vi "GUI_001.vi"(2 "Input":dbl) -> (0 "Slide":dbl(slide) scale=0.0..100.0)   [LabVIEW 2019]
doc: "This VI adds noise to user defined data"
uses:
  <vilib>/Analysis/baseanly.llb/Mean (DBL).vi
  <vilib>/Analysis/NI_AALBase.lvlib
panel:
  out "Histogram Graph":T1(graph)
  out "output data mean":dbl format="%0.2f"
  out "Output data":dbl[](array[numeric])
  in  "noise offset":dbl
  in  "noise gain":dbl
  in  "Operation Menu":T2(ring)
  out "Indicator":string
  in  "Control":string
  in  "stop":bool
  out "Waveform Chart":dbl(graph)
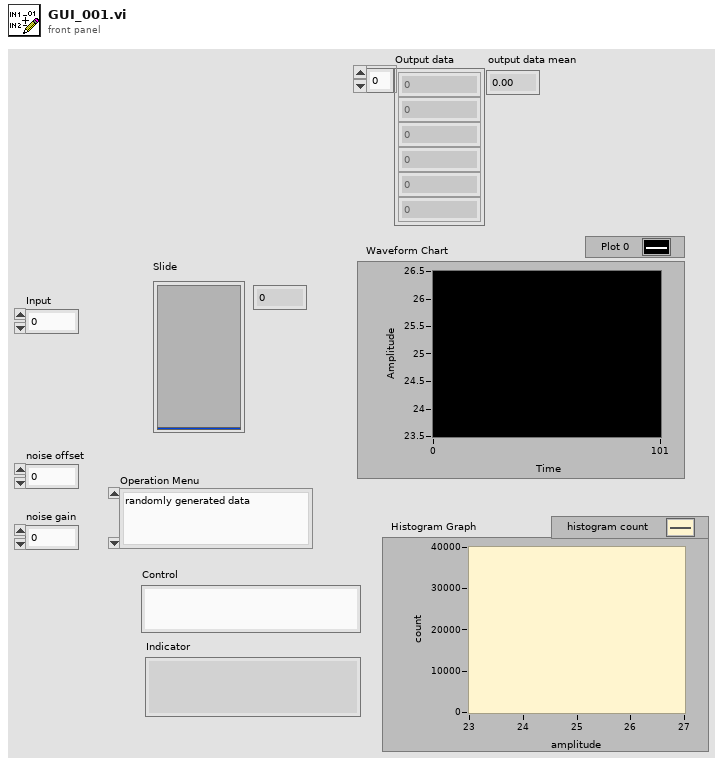
[diagram p1: front panel]
types:
  T1 = cluster{"X Values":dbl[], "Histogram: h(x)":i32[]}
  T2 = enum16{"randomly generated data", "user inserted data"}
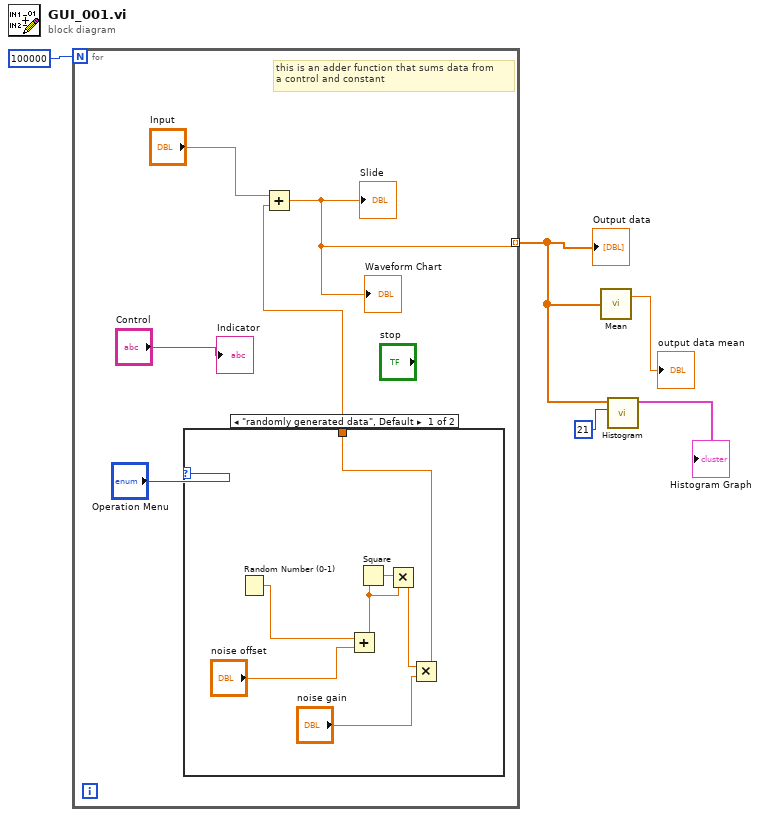
[diagram p0: block diagram]
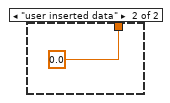
[diagram p2: hidden frame]
diagram:
  n1 = for {
    N: 100000 -> [_]
    tunnel: [w6] -> w3 mode=indexing
    # "this is an adder function that sums data from\na control and constant"
    n2 = case shown="\"randomly generated data\", Default" "Operation Menu" {
      tunnel: [w16 0.0] -> w7
      frame "randomly generated data", Default {
        n3 = Random Number (0-1)() -> (number: 0 to 1=w13:dbl)
        n4 = Add(x=w13, y="noise offset") -> (x+y=w12:dbl)
        n5 = Square(x=w12) -> (x^2=w15:dbl)
        n6 = Multiply(x=w15, y=w12) -> (x*y=w11:dbl)
        n7 = Multiply(x=w11, y="noise gain") -> (x*y=w16:dbl)
      }
      frame "user inserted data" {
      }
    }
    n8 = Add(x="Input", y=w7) -> (x+y=w6:dbl)
    "Slide" <- w6
    "Waveform Chart" <- w6
    "Indicator" <- "Control"
  }
  "Output data" <- w3
  n9 = call-poly <vilib>:"Mean.vi"("X"=w3) -> ("mean"=→"output data mean":dbl)  [unwired: 1 out]
  n10 = call <vilib>:"Histogram.vi"("intervals"=21, "X"=w3) -> ("Histogram Graph"=→"Histogram Graph":T1)  [unwired: 6 in, 3 out]
